vi "PostStop - Triaxial UU (SubVI).vi"(8 "error in (no error)":errorcluster, 11 "Cluster in in":T1 {"M Event" items=["Stop", "Running", "PID", "Up Limit", "Down Limit", "Load Limit"]; "Test Type" items=["Please Select", "Triaxial Shear", "Triaxial UU", "Shearbox", "Permeability", "Consolidation (Stepped Loading)/Swelling", "Saturation (Incremental)", "User Defined", "UCT", "Isotropic Consolidation", "Swelling Pressure"]; "Data"."Test Type" items=["Please Select", "Triaxial Shear", "Triaxial UU", "Shearbox", "Permeability", "Consolidation (Stepped Loading)/Swelling", "Saturation (Incremental)", "User Defined", "UCT", "Isotropic Consolidation", "Swelling Pressure"]}) -> (0 "error out":errorcluster, 2 "Enum":T10, 3 "Cluster out":T1 {"M Event" items=["Stop", "Running", "PID", "Up Limit", "Down Limit", "Load Limit"]; "Test Type" items=["Please Select", "Triaxial Shear", "Triaxial UU", "Shearbox", "Permeability", "Consolidation (Stepped Loading)/Swelling", "Saturation (Incremental)", "User Defined", "UCT", "Isotropic Consolidation", "Swelling Pressure"]; "Data"."Test Type" items=["Please Select", "Triaxial Shear", "Triaxial UU", "Shearbox", "Permeability", "Consolidation (Stepped Loading)/Swelling", "Saturation (Incremental)", "User Defined", "UCT", "Isotropic Consolidation", "Swelling Pressure"]})   [LabVIEW 2019]
uses:
  Controls/RunTest - State.ctl
  Controls/RunTest - Data Structure.ctl
  Controls/Test Panel - Data Structure.ctl
  Controls/Station - Test Type.ctl
  <vilib>/Utility/miscctls.llb/LVRowAndColumnTypeDef.ctl
  Controls/RunTest - Calculate Data.ctl
  <vilib>/httpClient/ClientHandle.ctl
  Controls/RunTest - Start Condition.ctl
  Controls/RunTest - Stop Condition.ctl
  Controls/UDP - Event.ctl
  Controls/UDP - Command.ctl
  <vilib>/httpClient/LabVIEWHTTPClient.lvlib
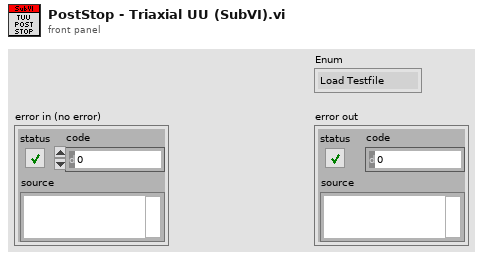
[diagram p1: front panel]
types:
  T1 = typedef "RunTest - Data Structure.ctl" = cluster{"Test Plan":string[], "PlanRow":i32, "Device Name":string[], "Timeout":i32, "Start?":bool, "Pause?":bool, "IP Address":string[], "LogRow":i32, "Logtype":u16, "Log Elapse":sgl, "Data":T2, "Stop log?":bool, "tdms":refnum<k34>, "Sensor Data":sgl[], "Start time":timestamp, "Prev Log Elapse":u32, "Plot":u16, "X-Axis":u16[], "Y-Axis":u16[], "XY":cluster{"X":dbl, "Y":dbl}[][], "End Stage?":bool, "1run":bool, "Condition":u16[], "Start Con":bool, "Log Con":bool, "Stop Con":bool, "Start Elapse":dbl, "Start Load":dbl, "Motor":i32, "StartRow":i32, "number log":i32, "Dir":bool, "Start time test":timestamp, "Auto":bool, "Check return?":bool, "Inv":cluster{"M":i32[], "Bool":bool[]}, "tdms temp":refnum<k34>, "Zero?":bool, "Plot Timer":dbl, "1st Run":bool, "TDMS Path":path, "MaxLoad":dbl, "Log Timer":sgl[], "Test Type":T3, "Log Sensor":string[], "Save?":bool, "1st Log":bool, "Y-Axis 2":u16[], "On Y-Axis 2":bool, "Decimal":u8[], "Init":cluster{"PWP TS":sgl, "Load TS":sgl, "Volume TS":sgl, "Disp TS":sgl, "CP":sgl, "Vol In":sgl, "Vol Out":sgl, "Load UCT":sgl, "Disp UCT":sgl, "PWP Sat":sgl, "CP Sat":sgl, "Volume IsoCons":sgl, "PWP IsoCons":sgl, "PWP TUU":sgl, "Load TUU":sgl, "Volume TUU":sgl, "Disp TUU":sgl, "Load Cons":sgl, "Disp Cons":sgl, "Volume Sat":sgl, "Vertical Load SB":sgl, "Vertical Disp SB":sgl, "H Disp SB":sgl, "H Load SB":sgl}, "Calc":T5, "Device Index":i32[], "Channel Index":i32[], "http ref":T6, "fileid":string, "Step Cons":cluster{"V Stress":sgl, "H Settlement":sgl}, "RunTest":bool, "Graph Last":i32, "Init?":bool, "Datalog":bool[], "Start":T7, "Stop":T8, "Running?":bool, "StartTime":dbl, "Log Prev Time":dbl, "KeyName":string[], "Test RunTime":dbl, "Log Prev Axial":dbl, "M Event":T9[], "Last Log":bool, "popup":bool, "PreStart UU":bool, "PreStart Sat":bool}
  T2 = typedef "Test Panel - Data Structure.ctl" = cluster{"Station":string, "Sample ID":string, "Job No":string, "Job Description":string, "Filename":string, "Test Type":T3, "Speciment No":string, "Depth":string, "Height":string, "Diameter/Length":string, "Weight":string, "Test Parameter":string, "Station[]":string[], "Edit Pos":T4, "Edit Pos Prev":T4, "Area":string, "Path":string}
  T3 = typedef "Station - Test Type.ctl" = u16
  T4 = typedef "LVRowAndColumnTypeDef.ctl" = cluster{"Row":i32, "Column":i32}
  T5 = typedef "RunTest - Calculate Data.ctl" = cluster{"TS":cluster{"Change PWP":sgl, "Change Vol":sgl, "Axial Load":sgl, "CiL":sgl, "Deviator":sgl, "Axial Strain":sgl, "MaxDeviator":sgl}, "TUU":cluster{"Change PWP":sgl, "Axial Load":sgl, "CiL":sgl, "Deviator":sgl, "Axial Strain":sgl, "MaxDeviator":sgl}, "Sat":cluster{"B Value":sgl, "PWP Diss":sgl, "CPP":sgl, "CV":sgl}, "Per":cluster{"Change Vol In":sgl, "Change Vol Out":sgl, "Mean Vol":sgl, "Gradient Pressure":sgl, "Outlet Flow":sgl, "Inlet Flow":sgl, "I X1":sgl, "I X2":sgl, "I Y1":sgl, "I Y2":sgl, "O X1":sgl, "O X2":sgl, "O Y1":sgl, "O Y2":sgl}, "Step Cons":cluster{"V Stress":sgl, "H Settlement":sgl, "Total H Settle":sgl, "Prev Total H":sgl}, "UCT":cluster{"ALC":sgl, "H Change":sgl, "Deviator":sgl, "Axial Strain":sgl, "V Stress":sgl, "MaxDeviator":sgl}, "ISO Cons":cluster{"CPP":sgl, "PWP Diss":sgl, "CV":sgl}, "SB":cluster{"Speci LenC":sgl, "Shear Strain":sgl, "H LC":sgl, "Normal Stress":sgl, "Shear Stress":sgl, "MaxShear":sgl}}
  T6 = typedef "LabVIEWHTTPClient.lvlib/ClientHandle.ctl" = refnum<k1>
  T7 = typedef "RunTest - Start Condition.ctl" = cluster{"Cons":cluster{"VS":dbl, "Delay":bool, "No Delay":dbl}, "Sat":cluster{"CP":dbl, "BP":dbl, "StartBP":bool, "Target CP":bool, "Target BP":bool}, "Iso":cluster{"Select":dbl, "BP":dbl, "IC2":dbl, "IC3":dbl, "IC4":dbl, ". IC6":bool, "IC6":dbl, "IC6-2":dbl, "Target":bool, "Time Cond":dbl, "Last PWP":dbl}, "TS":cluster{"SS":dbl, "Engage":bool, "ES":dbl, "LC":dbl, "PreStart":bool, "Trig SS":bool, "Drain":dbl}, "TUU":cluster{"SS":dbl, "Engage":bool, "ES":dbl, "LC":dbl, "PreStart":bool, "Trig SS":bool, "CP":dbl, "Delay Value":dbl, "Delay":bool, "CP PID":bool}, "UCT":cluster{"SS":dbl, "Engage":bool, "ES":dbl, "LC":dbl, "PreStart":bool, "Trig SS":bool}, "Enable?":bool, "SB":cluster{"SS":dbl, "Engage":bool, "ES":dbl, "LC":dbl, "PreStart":bool, "Trig SS":bool, "VS":dbl, "Delay Value":dbl, "Delay":bool, "VS PID":bool}, "Perm":cluster{"DP":dbl}}
  T8 = typedef "RunTest - Stop Condition.ctl" = cluster{"Cons":cluster{"Select":i32, "Disp":dbl, "Time":dbl, "Time2":dbl, "Disp 2":dbl, "Time Cond":dbl, "Last Disp":dbl, "Swell":bool}, "Sat":cluster{"Select":i32, "PP":dbl, "Time":dbl, "VC":dbl, "Time2":dbl, "Time Cond":dbl, "Last PP":dbl, ".B":bool, "B":dbl, "Last Vc":dbl, "Time Cond 2":dbl, "Time3":dbl, "Time Cond 3":dbl, "B Achieve":bool}, "Iso":cluster{"PP":dbl, "Time":dbl, "VC":dbl, "Time2":dbl, "Time Cond":dbl, "Last Vc":dbl, ".PP":bool, "Time Cond 2":dbl, "Select":i32}, "TS":cluster{"Axial":dbl, ".MaxDev":bool, "MaxDev Value":dbl, "Return":bool, "Reset":bool, "Prev Time":dbl, "PostStop Run":bool, "CP Stop":bool, "BP Stop":bool, "PostStop Trig":bool, "Reset Value":dbl, "BPTrig":bool, "CPTrig":bool, "VLCTrig":bool}, "TUU":cluster{"Axial":dbl, ".MaxDev":bool, "MaxDev Value":dbl, "Return":bool, "Reset":bool, "Prev Time":dbl, "PostStop Run":bool, "CP Stop":bool, "BP Stop":bool, "PostStop Trig":bool, "Reset Value":dbl, "BPTrig":bool, "CPTrig":bool, "VLCTrig":bool}, "UCT":cluster{"Axial":dbl, ".MaxDev":bool, "MaxDev Value":dbl, "Return":bool, "Reset":bool, "Prev Time":dbl, "PostStop Run":bool, "CP Stop":bool, "BP Stop":bool, "PostStop Trig":bool}, "Enable?":bool, "SB":cluster{"Shear":dbl, ".MaxShear":bool, "MaxShear Value":dbl, "Return":bool, "Reset":bool, "Prev Time":dbl, "PostStop Run":bool, "CP Stop":bool, "BP Stop":bool, "PostStop Trig":bool, "Reset Value":dbl, "BPTrig":bool, "CPTrig":bool, "VLCTrig":bool}, "Perm":cluster{"Max Time":bool, "Reset":bool, "PostStop Run":bool, "Ratio":bool, "Reset Value":dbl, "Time":dbl, "RatioTime":dbl, "RatioMore":dbl, "RatioLess":dbl, "Time Cond":dbl, "Time Cond 2":dbl, "Prev IF":dbl, "Prev OF":dbl, "PostStop Trig":bool, "BP Trig":bool, "DP Stop":bool, "BP Stop":bool, "CP Stop":bool, "CP Trig":bool}, "SP":cluster{".Max Time":bool, ".Time":bool, "Time":dbl, "MaxTime":dbl, "Time Cond":dbl, "Max Time Cond":dbl, "Stress":dbl}}
  T9 = typedef "UDP - Event.ctl" = u16
  T10 = typedef "RunTest - State.ctl" = enum16{"Load Testfile", "Notifier", "Init", "Idle", "Load", "Read DB", "Run", "Pause", "Stop", "Check Start", "Check Stop", "Check Post Stop", "Check Log", "EndStage", "Data View", "Display", "Graph", "Graph Old", "Close", "Stop PID", "Check Limit", "Auto", "Up", "Log", "Zero", "Machine Control", "Save Report"}
  T11 = typedef "UDP - Command.ctl" = enum16{"Stop", "Jog Up", "Jog Down", "Ramp Up", "Ramp Down", "PID Target", "PID Ramp", "Disp Run", "Read Ch Data", "Zero Channel", "Zero Disp", "Read Sensor", "Write Sensor", "Read ADC", "Write ADC", "Read PID", "Write PID", "Read Test", "Write Test", "Read System", "Write System", "Read Datalog", "Read Datalog Sensor"}
  T12 = cluster{"Target Load":sgl, "Target Disp":sgl, "Rate":sgl, "Speed":sgl}
  T13 = enum16{"None", "Run Target", "Run Ramp", "Run Disp"}
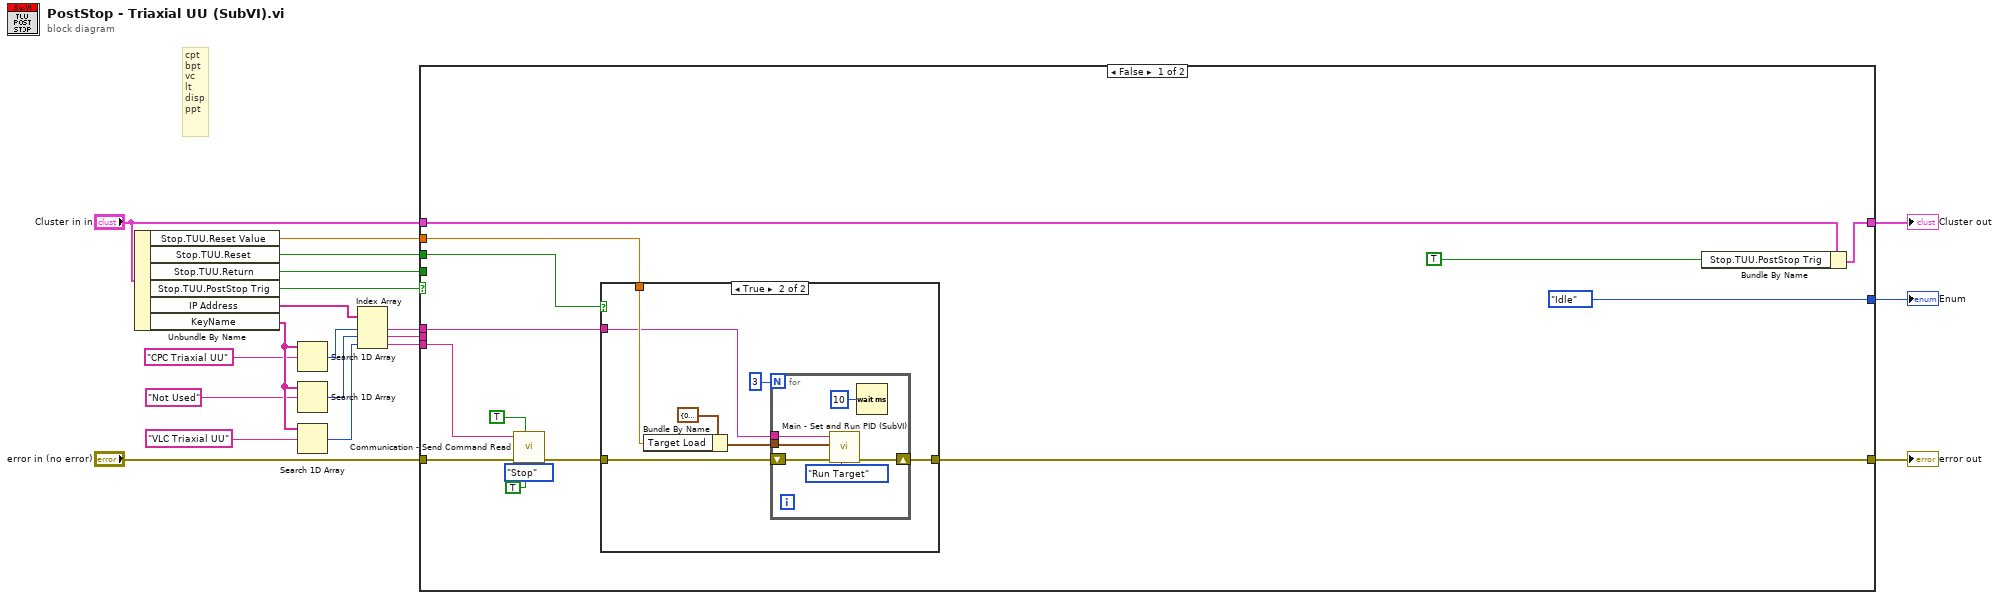
[diagram p0: block diagram]
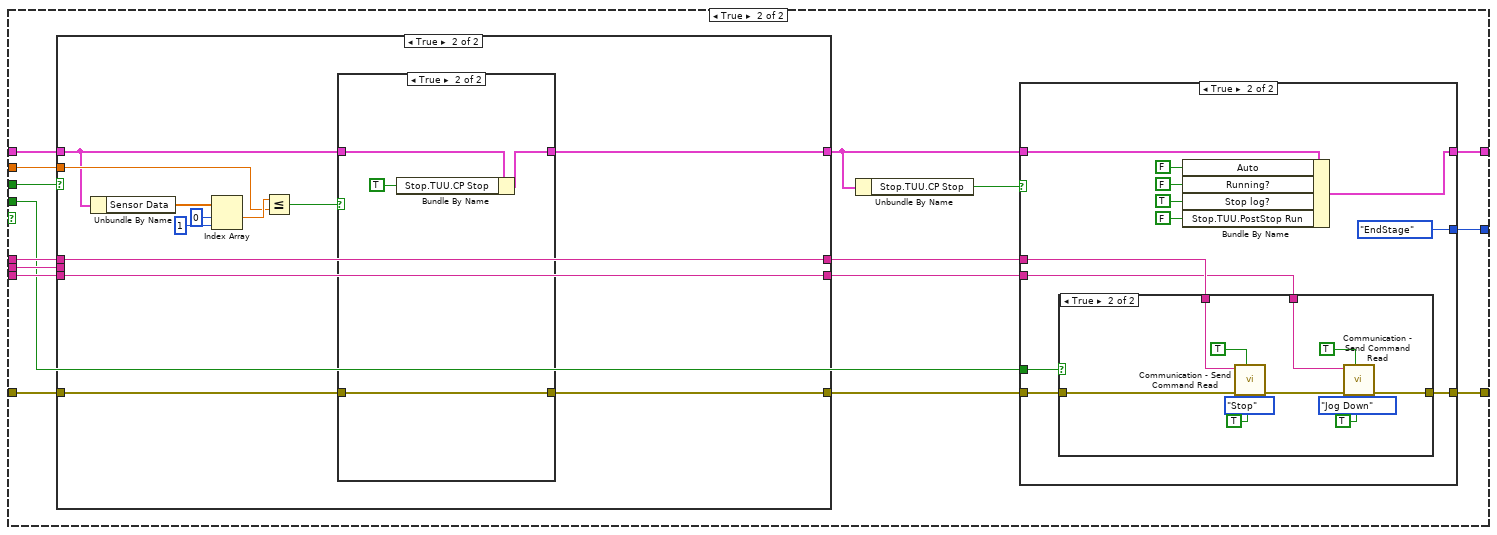
[diagram p3: hidden frame]
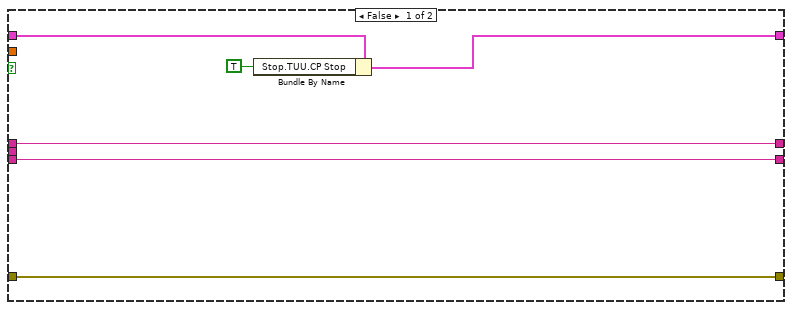
[diagram p4: hidden frame]
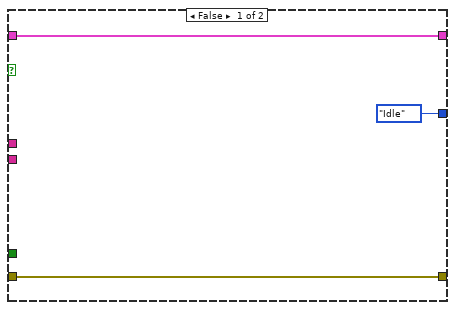
[diagram p6: hidden frame]
diagram:
  # "cpt\nbpt\nvc\nlt\ndisp\nppt"
  n1 = Unbundle By Name("Cluster in in") -> ("Stop.TUU.Reset Value"=w20:dbl, "Stop.TUU.Reset"=w18:bool, "Stop.TUU.Return"=w17:bool, "Stop.TUU.PostStop Trig"=w2:bool, "IP Address"=w19:string[], "KeyName"=w15:string[])
  n2 = Search 1D Array(1D array=w15, element="CPC Triaxial UU" ("String")) -> (index of element=w8:i32)  [unwired: 1 in]
  n3 = Search 1D Array(1D array=w15, element="Not Used" ("String")) -> (index of element=w9:i32)  [unwired: 1 in]
  n4 = Search 1D Array(1D array=w15, element="VLC Triaxial UU" ("String")) -> (index of element=w14:i32)  [unwired: 1 in]
  n5 = Index Array(array=w19, index #1=w8, index #2=w9, index #3=w14) -> (element #1=w10:string, element #2=w11:string, element #3=w16:string)
  n6 = case shown="False" w2 {
    tunnel: [w31 w59] -> w3
    tunnel: "Cluster in in" -> [w33 w60]
    tunnel: [w21 w57] -> w5
    tunnel: "error in (no error)" -> [w25 w64]
    tunnel: w10 -> [w34 w63]
    tunnel: w11 -> [_ w62]
    tunnel: [RunTest_-_State."Idle" w61] -> w12
    tunnel: w16 -> [w24 w53]
    tunnel: w17 -> [_ w51]
    tunnel: w18 -> [w29 w49]
    tunnel: w20 -> [w22 w55]
    frame False {
      n7 = call "Communication - Send Command Read.vi"("Fron?"=TRUE, "Bypass?"=TRUE, "error in (no error)"=w25, "Action"=UDP_-_Command."Stop", "Device IP Address"=w24) -> ("error out"=w23:errorcluster)  [unwired: 6 in]
      n8 = case shown="True" w29 {
        tunnel: w23 -> [w35 w40]
        tunnel: w34 -> [_ w37]
        tunnel: [w35 w38] -> w21
        tunnel: w22 -> [_ w39]
        frame False {
        }
        frame True {
          n9 = Bundle By Name(cluster=T12 {"Target Load"=0.0, "Target Disp"=0.0, "Rate"=0.0, "Speed"=0.0} ("Test"), "Target Load"=w39) -> (w41:T12)
          n10 = for {
            N: 3 -> [_]
            tunnel: w41 -> [w47]
            tunnel: w37 -> [w44]
            shift-right: [w45] -> w38
            shift-left: w40 -> [w46]
            n11 = call "Main - Set and Run PID (SubVI).vi"("Action"=T13."Run Target", "error in (no error)"=w46, "Test"=w47, "IP Address"=w44) -> ("error out"=w45:errorcluster)  [unwired: 7 in]
            n12 = Wait (ms)(milliseconds to wait=u32 10) -> ()  [unwired: 1 out]
          }
        }
      }
      n13 = Bundle By Name(cluster=w33, "Stop.TUU.PostStop Trig"=TRUE ("Stop.TS.PostStop Run")) -> (w31:T1)
    }
    frame True {
      n14 = case shown="True" w49 {
        tunnel: w64 -> [w67 w71]
        tunnel: w63 -> [w66 w74]
        tunnel: w62 -> [_ _]
        tunnel: w60 -> [w69 w72]
        tunnel: [w68 w82] -> w58
        tunnel: [w67 w81] -> w56
        tunnel: w55 -> [_ w75]
        tunnel: [w66 w74] -> w54
        tunnel: w53 -> [w65 w73]
        tunnel: [w65 w73] -> w52
        frame False {
          n15 = Bundle By Name(cluster=w69, "Stop.TUU.CP Stop"=TRUE ("Stop.TS.CP Stop")) -> (w68:T1)
        }
        frame True {
          n16 = Unbundle By Name(w72) -> ("Sensor Data"=w80:sgl[])
          n17 = Index Array(array=w80, index #1=0 ("index"), index #2=1 ("index")) -> (element #1=w77:sgl)  [unwired: 1 out]
          n18 = Less Or Equal?(x=w77, y=w75) -> (x <= y?=w76:bool)
          n19 = case shown="True" w76 {
            tunnel: w71 -> [w84 w85]
            tunnel: [w84 w85] -> w81
            tunnel: w72 -> [w83 w87]
            tunnel: [w83 w86] -> w82
            frame False {
            }
            frame True {
              n20 = Bundle By Name(cluster=w87, "Stop.TUU.CP Stop"=TRUE ("Stop.TS.BP Stop")) -> (w86:T1)
            }
          }
        }
      }
      n21 = Unbundle By Name(w58) -> ("Stop.TUU.CP Stop"=w50:bool)
      n22 = case shown="True" w50 {
        tunnel: [RunTest_-_State."Idle" RunTest_-_State."EndStage"] -> w61
        tunnel: [w90 w100] -> w59
        tunnel: w58 -> [w90 w102]
        tunnel: [w89 w95] -> w57
        tunnel: w56 -> [w89 w97]
        tunnel: w54 -> [_ w96]
        tunnel: w52 -> [_ w94]
        tunnel: w51 -> [_ w93]
        frame False {
        }
        frame True {
          n23 = case shown="True" w93 {
            tunnel: w97 -> [w104 w105]
            tunnel: w96 -> [_ w112]
            tunnel: [w104 w107] -> w95
            tunnel: w94 -> [_ w106]
            frame False {
            }
            frame True {
              n24 = call "Communication - Send Command Read.vi"("Fron?"=TRUE, "Bypass?"=TRUE, "error in (no error)"=w105, "Action"=UDP_-_Command."Stop", "Device IP Address"=w112) -> ("error out"=w108:errorcluster)  [unwired: 6 in]
              n25 = call "Communication - Send Command Read.vi"("Fron?"=TRUE, "Bypass?"=TRUE, "error in (no error)"=w108, "Action"=UDP_-_Command."Jog Down", "Device IP Address"=w106) -> ("error out"=w107:errorcluster)  [unwired: 6 in]
            }
          }
          n26 = Bundle By Name(cluster=w102, "Auto"=FALSE, "Running?"=FALSE, "Stop log?"=TRUE, "Stop.TUU.PostStop Run"=FALSE) -> (w100:T1)
        }
      }
    }
  }
  "Enum" <- w12
  "error out" <- w5
  "Cluster out" <- w3
